vi "Main_4_Dynamic_9239[FPGA].vi"() -> ()   [LabVIEW 2017]
uses:
  <vilib>/LabVIEW Targets/FPGA/cRIO/shared/nicrio_ModuleControls/nicrio_cRIO-9232_ConfigModeRing.ctl
  <vilib>/rvi/Emulation/niFpgaGetClockAttributes.vi
  <vilib>/rvi/Emulation/niFpgaSctlEmulationGetInTimedLoop.vi
  <vilib>/rvi/Emulation/niFpgaEmulationReportErrorSimple.vi
  <vilib>/rvi/Emulation/niFpgaProcessEmulError.vi
  <vilib>/rvi/eio/common/nirviEmuTemplateMethod_errors.vi
  <vilib>/rvi/interface/RandomDataEmulation/niFpgaRandomDataHandleErrors.vi
  <vilib>/rvi/Emulation/niFpgaCriticalErrorInLSC.vi
  <vilib>/eio/EIONode/EIONode.xnode
  <vilib>/rvi/DataTransferAndStorage/Container/XNode/niFpgaContainer.xnode
  <vilib>/rvi/interface/RandomDataEmulation/nirviRandomDataFpgaReadWriteTemplate.vi
  <vilib>/addons/InsightCM/Devices/Shared/Cms/Fpga/Acquisition/source/subVIs/VibAPI_4/BOP_VibAPI_4.lvlib
panel:
  out "Chassis Temperature":sgl
  in  "Custom Scale Intercept":sgl[](array[numeric])=[0.0, 0.0, 0.0, 0.0, 0.0, 0.0, 0.0, 0.0, 0.0, 0.0, 0.0, 0.0, 0.0, 0.0, 0.0, 0.0, 0.0, 0.0, 0.0, 0.0, 0.0, 0.0, 0.0, 0.0, 0.0, 0.0, 0.0, 0.0, 0.0, 0.0, 0.0, 0.0]
  out "FPGA Error":errorcluster
  out "Finished":bool
  in  "Stop":bool
  out "Module Underflow":bool
  out "DMA FIFO Full":bool
  out "Chan Count":bool
  out "Acq Loop Ticks":u32
  out "Short Circuit Chan Array":bool[](array[boolean])
  out "Open Loop Chan Array":bool[](array[boolean])
  out "First Read":bool
  in  "Total Avail Channels":i32=4
  in  "Data Rate [S/s]":u32=1280
  in  "Custom Scale Slope":sgl[](array[numeric])=[0.0, 0.0, 0.0, 0.0, 0.0, 0.0, 0.0, 0.0, 0.0, 0.0, 0.0, 0.0, 0.0, 0.0, 0.0, 0.0, 0.0, 0.0, 0.0, 0.0, 0.0, 0.0, 0.0, 0.0, 0.0, 0.0, 0.0, 0.0, 0.0, 0.0, 0.0, 0.0]
  in  "Acquisition Type":enum16{"Finite Samples", "Continuous Samples"}(ring)
  in  "Samps per Chan [Finite]":i32=5120
  in  "Input Config Array":T1[](array[typedef])=[0, 0, 0, 0, 0, 0, 0, 0, 0, 0, 0, 0, 0, 0, 0, 0, 0, 0, 0, 0, 0, 1, 1, 1, 0, 0, 0, 0, 0, 0, 0, 0] items=["AC Coupled", "DC Coupled", "IEPE AC Coupled"]
  in  "Number of Modules":i16=1
  in  "Enable Chan Array":bool[](array[boolean])=[FALSE, FALSE, FALSE, FALSE, FALSE, FALSE, FALSE, FALSE, FALSE, FALSE, FALSE, FALSE, FALSE, FALSE, FALSE, FALSE, FALSE, FALSE, FALSE, FALSE, FALSE, FALSE, FALSE, FALSE, FALSE, FALSE, FALSE, FALSE, FALSE, FALSE, FALSE, FALSE]
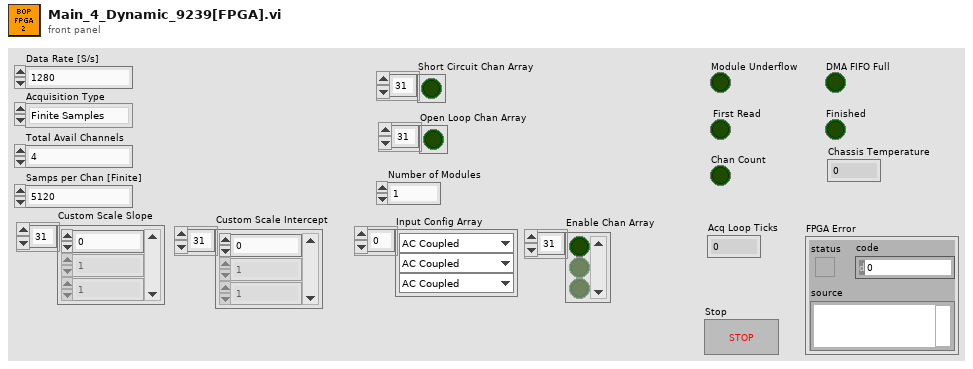
[diagram p1: front panel]
types:
  T1 = typedef "nicrio_cRIO-9232_ConfigModeRing.ctl" = u8
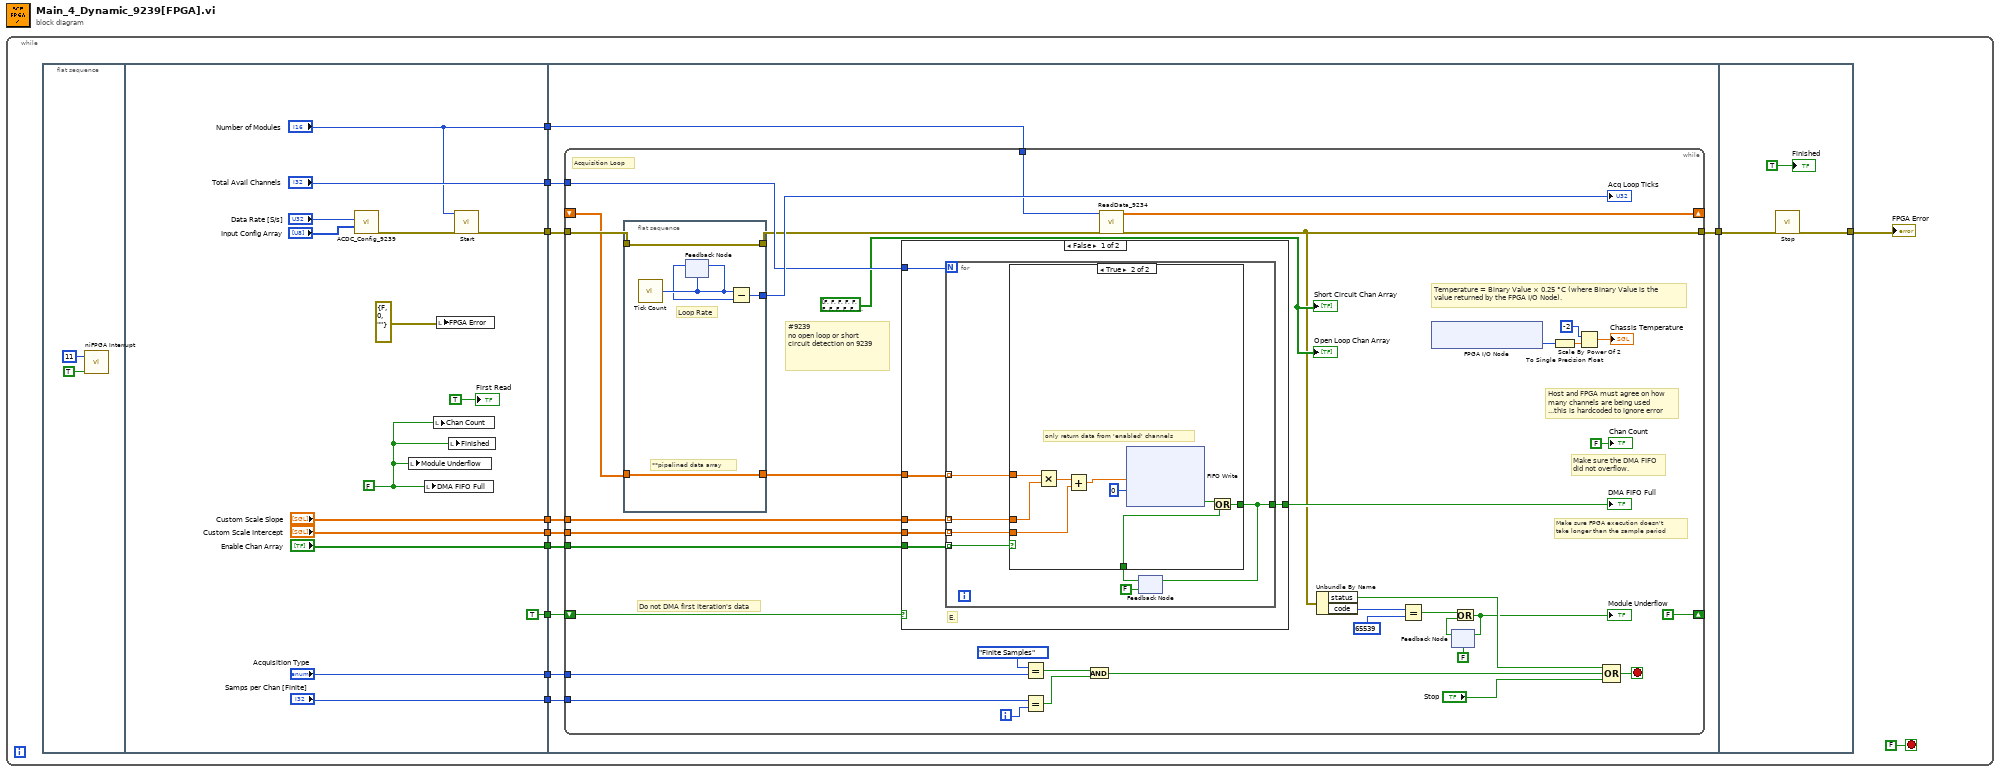
[diagram p0: block diagram]
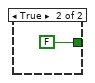
[diagram p3: hidden frame]
diagram:
  n1 = while {
    stop <- FALSE stop-if-true
    n2 = flat-sequence {
      tunnel: [w18] -> w11
      tunnel: ["Custom Scale Slope"] -> w10
      tunnel: ["Acquisition Type"] -> w9
      tunnel: ["Samps per Chan [Finite]"] -> w8
      tunnel: ["Total Avail Channels"] -> w7
      tunnel: [TRUE ("t")] -> w6
      tunnel: ["Number of Modules"] -> w4
      tunnel: ["Enable Chan Array"] -> w3
      tunnel: ["Custom Scale Intercept"] -> w1
      tunnel: w11 -> [w38]
      tunnel: w10 -> [w37]
      tunnel: w9 -> [w35]
      tunnel: w8 -> [w34]
      tunnel: w7 -> [w39]
      tunnel: w6 -> [w36]
      tunnel: [w33] -> w5
      tunnel: w4 -> [w32]
      tunnel: w3 -> [w31]
      tunnel: w1 -> [w30]
      tunnel: w5 -> [w107]
      tunnel: [w106] -> w2
      frame #0 {
        n3 = call <vilib>:"niFPGA Interrupt.vi"("Wait Until Cleared (F)"=TRUE ("Wait Until Cleared"), "IRQ Number (0)"=u8 11 ("IRQ Number")) -> ()  [unwired: 1 in]
      }
      frame #1 {
        w23 = FALSE ("Module Underflow")
        n4 = call <vilib>:"ACDC_Config_9239.vi"("Input Config Array"="Input Config Array", "Data Rate [S/s]"="Data Rate [S/s]") -> ("error out"=w15:errorcluster)  [unwired: 9 in]
        n5 = local write "Module Underflow"(w23) -> ()
        n6 = local write "DMA FIFO Full"(w23) -> ()
        n7 = local write "Chan Count"(w23) -> ()
        n8 = local write "FPGA Error"(errorcluster {"status"=FALSE, "code"=0, "source"=""} ("FPGA Error")) -> ()
        n9 = local write "Finished"(w23) -> ()
        n10 = call <vilib>:"Start.vi"("error in (no error)"=w15, "Module Config Selector"="Number of Modules") -> ("error out"=w18:errorcluster)  [unwired: 9 in]
        "First Read" <- TRUE ("First Read")
      }
      frame #2 {
        n11 = while {
          tunnel: w38 -> [w70]
          tunnel: [w40] -> w33
          tunnel: w35 -> [w72]
          tunnel: w34 -> [w71]
          shift-right: [w41] -> _
          shift-left: _ -> [w68]
          tunnel: w39 -> [w52]
          tunnel: w37 -> [w51]
          shift-right: [FALSE ("t")] -> _
          shift-left: w36 -> [w55]
          tunnel: w32 -> [w42]
          tunnel: w31 -> [w50]
          tunnel: w30 -> [w49]
          i -> [w66]
          stop <- w75 stop-if-true
          w44 = bool[] [FALSE, FALSE, FALSE, FALSE, FALSE, FALSE, FALSE, FALSE, FALSE, FALSE, FALSE, FALSE, FALSE, FALSE, FALSE, FALSE, FALSE, FALSE, FALSE, FALSE, FALSE, FALSE, FALSE, FALSE, FALSE, FALSE, FALSE, FALSE, FALSE, FALSE, FALSE, FALSE] ("Short Circuit Chan Array")
          # "#9239\nno open loop or short circuit detection on 9239"
          # "Temperature = Binary Value × 0.25 °C (where Binary Value is the value returned by the FPGA I/O Node)."
          # "Do not DMA first iteration's data"
          # "Acquisition Loop"
          # "Host and FPGA must agree on how \nmany channels are being used\n...this is hardcoded to ignore error"
          # "Make sure the DMA FIFO\ndid not overflow."
          # "Make sure FPGA execution doesn't\ntake longer than the sample period"
          n12 = flat-sequence {
            tunnel: [w105] -> w43
            tunnel: w70 -> [w105]
            tunnel: [w102] -> w69
            tunnel: w68 -> [w101]
            tunnel: [w101] -> w53
            frame #0 {
              # "**pipelined data array"
              # "Loop Rate"
              n13 = call "Tick Count"() -> ("Tick Count(Ticks)"=w104:u32)
              n14 = feedback-in #1(w104) -> ()
              n15 = feedback #1(w104) -> (w103:u32)
              n16 = Subtract(x=w104, y=w103) -> (x-y=w102:u32)
            }
          }
          n17 = case shown="False" w55 {
            tunnel: [w82 FALSE] -> w54
            tunnel: w51 -> [w81 _]
            tunnel: w53 -> [w80 _]
            tunnel: w52 -> [w79 _]
            tunnel: w50 -> [w78 _]
            tunnel: w49 -> [w77 _]
            frame False {
              # "E."
              n18 = for {
                N: w79 -> [_]
                tunnel: [w88] -> w82
                tunnel: w80 -> [w87] mode=indexing
                tunnel: w81 -> [w86] mode=indexing
                tunnel: w78 -> [w84] mode=indexing
                tunnel: w77 -> [w83] mode=indexing
                n19 = feedback #2(FALSE) -> (w89:bool)
                n20 = case shown="True" w84 {
                  tunnel: w89 -> [w90 w99]
                  tunnel: [w90 w98] -> w88
                  tunnel: w87 -> [_ w97]
                  tunnel: w86 -> [_ w96]
                  tunnel: w83 -> [_ w91]
                  frame False {
                  }
                  frame True {
                    # "only return data from 'enabled' channels"
                    n21 = Multiply(x=w97, y=w96) -> (x*y=w93:sgl)
                    n22 = Add(x=w93, y=w91) -> (x+y=w92:sgl)
                    n23 = xnode ("FIFO Write")("Element"=w92, "Timeout"=0) -> ("Timed Out?"=w94:bool)  [unwired: 1 in, 1 out]
                    n24 = Or(x=w94, y=w99) -> (x .or. y?=w98:bool)
                  }
                }
                n25 = feedback-in #2(w88) -> ()
              }
            }
            frame True {
            }
          }
          "DMA FIFO Full" <- w54
          n26 = Equal?(x=enum16{"Finite Samples", "Continuous Samples"}."Finite Samples" ("y"), y=w72) -> (x = y?=w60:bool)
          n27 = Equal?(x=w71, y=w66) -> (x = y?=w59:bool)
          n28 = And(x=w60, y=w59) -> (x .and. y?=w58:bool)
          n29 = call <vilib>:"ReadData_9234.vi"("error in"=w43, "Module Config Selector"=w42) -> ("error out"=w40:errorcluster, "Data Array"=w41:sgl[])  [unwired: 8 in]
          n30 = Unbundle By Name(w40) -> ("status"=w65:bool, "code"=w73:i32)
          n31 = Equal?(x=w73, y=65539) -> (x = y?=w62:bool)
          n32 = xnode "FPGA I/O Node"() -> ("Chassis Temperature"=w46:i16)  [unwired: 1 in, 1 out]
          n33 = feedback #3(FALSE) -> (w64:bool)
          n34 = Or(x=w62, y=w64) -> (x .or. y?=w61:bool)
          "Module Underflow" <- w61
          n35 = feedback-in #3(w61) -> ()
          n36 = To Single Precision Float(number=w46) -> (single precision float=w48:sgl)
          n37 = Scale By Power Of 2(n=i16 -2, x=w48) -> (x*2^n=→"Chassis Temperature":sgl)
          n38 = Compound Arithmetic op=OR(w65, w58, "Stop") -> (w75:bool)
          "Chan Count" <- FALSE ("Chan Count")
          "Acq Loop Ticks" <- w69
          "Short Circuit Chan Array" <- w44
          "Open Loop Chan Array" <- w44
        }
      }
      frame #3 {
        n39 = call <vilib>:"Stop.vi"("error in (no error)"=w107) -> ("error out"=w106:errorcluster)  [unwired: 10 in]
        "Finished" <- TRUE ("Finished")
      }
    }
    "FPGA Error" <- w2
  }
